vi "Increment Counter.vi"(8 "error in":errorcluster) -> (0 "error out":errorcluster)   [LabVIEW 2014]
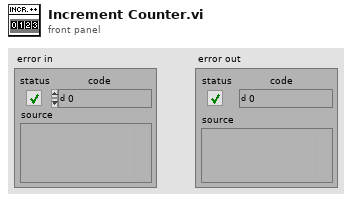
[diagram p1: front panel]
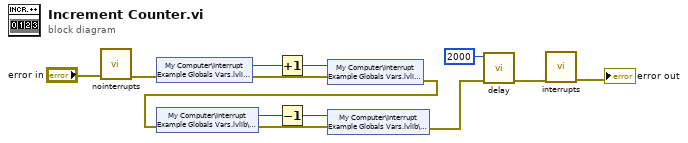
[diagram p0: block diagram]
diagram:
  n1 = call <vilib>:"nointerrupts.vi"("Error In"="error in") -> ("Error Out"=w11:errorcluster)  [unwired: 10 in]
  n2 = shared-variable "My Computer\\Interrupt Example Globals Vars.lvlib\\intCounter"(error in=w11) -> (w7:i32, error out=w13:errorcluster)
  n3 = Increment(x=w7) -> (x+1=w6:i32)
  n4 = shared-variable "My Computer\\Interrupt Example Globals Vars.lvlib\\intCounter"(w6, error in=w13) -> (error out=w2:errorcluster)
  n5 = shared-variable "My Computer\\Interrupt Example Globals Vars.lvlib\\intCounter2"(error in=w2) -> (w4:i32, error out=w3:errorcluster)
  n6 = Decrement(x=w4) -> (x-1=w5:i32)
  n7 = shared-variable "My Computer\\Interrupt Example Globals Vars.lvlib\\intCounter2"(w5, error in=w3) -> (error out=w1:errorcluster)
  n8 = call <vilib>:"delay.vi"("Error In"=w1, "time (ms)"=2000) -> ("Error Out"=w9:errorcluster)  [unwired: 9 in]
  n9 = call <vilib>:"interrupts.vi"("Error In"=w9) -> ("Error Out"=→"error out":errorcluster)  [unwired: 10 in]
